vi "Main.vi"() -> ()   [LabVIEW 2017]
doc: "This Continuous Measurement sample project is based on the Queued Message Handler template.\n\nThe Event Handling Loop generates messages based on user interface actions.\n\nThe Message Handling Loop processes messages generated by the Event Handling Loop, or by other messages. There are also Acquisition and Logging message handling loop subVIs, and a chart updating loop."
uses:
  controls/UI Data.ctl
  support/libs/PMU Buffer/Buffer DATA cluster.ctl
  controls/UI State.ctl
  acquisition/Acquisition Settings.ctl
  acquisition/Acquisition State.ctl
  logging/Logging Configuration.ctl
  logging/Logging State.ctl
  support/libs/PMU Buffer/Buffer Settings.ctl
  processing/Processing Settings.ctl
  controls/Acquired Data.ctl
  <vilib>/Utility/error.llb/DialogType.ctl
  support/libs/PMU Buffer/Buffer state.ctl
  b850246f-c621-4cc8-8cdb-6c63488b8d16.vi
  d6c7b380-5ef8-42a0-a533-ce26cb609579.vi
  5953c9e4-e6ed-48ce-a3e3-f4074e595e54.vi
  308fbb3a-e3c1-4651-8528-14e79cd65b6c.vi
  e1cf4c14-b580-4597-8acf-5221adc64a8a.vi
  17f702fa-b3ef-4227-89b6-1808d4fdff79.vi
  <vilib>/S3DK/PMU Recorder Light/PRL Channel Selector.vi
  support/settings/Get Config File Path.vi
  <vilib>/Utility/xml.llb/Read From XML File.vi
  <vilib>/Utility/xml.llb/Read From XML File(string).vi
  <vilib>/Utility/xml.llb/Write to XML File.vi
  <vilib>/Utility/xml.llb/Write to XML File(string).vi
  <vilib>/Utility/error.llb/Error Cluster From Error Code.vi
  <vilib>/ErrorRing/Error Ring.xnode
  Acquisition/Acquisition.lvlib
  Logging/Logging.lvlib
  support/User Event - Stop/User Event - Stop.lvlib
  support/Message Queue/Message Queue.lvlib
  support/settings/Settings Dialog.vi
  support/settings/Settings.lvlib
  processing/Processing.lvlib
  support/libs/PMU Buffer/PMU data buffer.lvlib
  <vilib>/S3DK/PMU Recorder Light/PMU Recorder Light.lvlib
panel:
  in  "Data Selector":bool
  in  "PRL Visible":bool
  out "Processing":bool=TRUE
  out "Display":bool
  out "Acquisition":bool=TRUE
  out "Events":bool=TRUE
  out "Buffer":bool
  out "UI Control":bool
  out "Waveform Chart":dbl[](graph)
  in  "Settings":bool
  in  "Start":bool
  in  "Stop":bool
  out "Status":string
  in  "Exit":bool
  # "Continuous Measurement Data Logger"
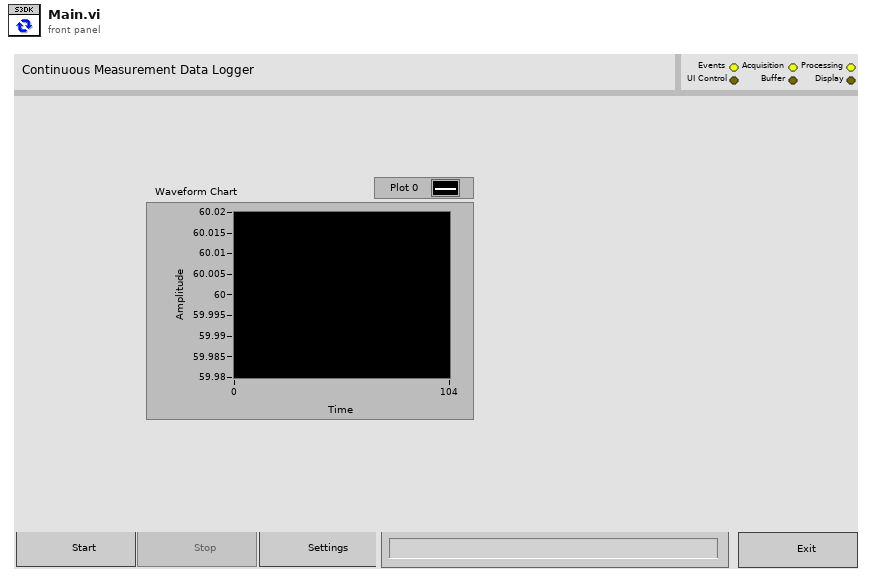
[diagram p1: front panel]
types:
  T1 = typedef "Acquired Data.ctl" = cluster{"Data":dbl[]}
  T2 = typedef "Processing.lvlib/Processing Settings.ctl" = cluster{"Settings":string, "Parameters":T3}
  T3 = typedef "PMU data buffer.lvlib/Buffer Settings.ctl" = cluster{"Index":i32, "Size":i32, "Samples":i32, "Ordered ?":bool}
  T4 = typedef "Logging.lvlib/Logging Configuration.ctl" = cluster{"Logging State":T5, "Settings":string, "Buffer":T3}
  T5 = typedef "Logging.lvlib/Logging State.ctl" = enum16{"Idle", "Logging"}
  T6 = typedef "Acquisition.lvlib/Acquisition Settings.ctl" = cluster{"Acquisition State":T7, "Settings":string, "Status":cluster{"Buffer":bool, "Config":bool, "Connect":bool}, "S3DK":cluster{"Signals":cluster{"Phasor":string[], "Analog":string[], "Digital":string[]}}}
  T7 = typedef "Acquisition.lvlib/Acquisition State.ctl" = enum16{"Idle S3DK", "Acquiring S3DK", "Idle CSV", "Acquiring CSV"}
  T8 = typedef "UI State.ctl" = enum16{"Idle", "Acquiring and Logging", "Waiting for Exit", "Waiting for Exit (Acq Stopped)", "Waiting for Exit (Log Stopped)", "Waiting for Stop", "Waiting for Stop (Acq Stopped)", "Waiting for Stop (Log Stopped)"}
  T9 = typedef "PMU data buffer.lvlib/Buffer DATA cluster.ctl" = cluster{timestamp, csg[], sgl[]}
  T10 = typedef "UI Data.ctl" = cluster{"Start Ref":refnum<vi>, "Stop Ref":refnum<vi>, "Settings Ref":refnum<vi>, "Exit Ref":refnum<vi>, "Status Ref":refnum<vi>, "Data Ref":refnum<vi>}
  T11 = cluster{"notifier out":refnum<notifier>, "notifier out":refnum<notifier>, "notifier out":refnum<notifier>}
  T12 = typedef "Message Queue.lvlib/All Message Queues.ctl" = cluster{"UI":refnum<queue>, "Acquisition":refnum<queue>, "Logging":refnum<queue>, "Processing":refnum<queue>}
  T13 = cluster{"Data Cluster":T6, "Logging Configuration":T4, "Processing Settings":T2}
  T14 = typedef "Settings.lvlib/Settings.ctl" = cluster{"Hardware Configuration":T6, "Logging Configuration":T4, "Processing Settings":T2}
  T15 = typedef "DialogType.ctl" = u16
  T16 = enum16{"Run", "Startup", "Get Status", "Pause", "Continue", "Shutdown", "Abort", "Open Panel", "Close Panel"}
  T17 = enum32{"Invalid", "Standard", "Closed", "Hidden", "Minimized", "Maximized"}
  T18 = typedef "PMU data buffer.lvlib/Buffer state.ctl" = enum16{"Init", "Change Size", "Flush", "Exit", "Add", "Get", "Hist_Toggle", "Add_Serv"}
  T19 = typedef "PMU data buffer.lvlib/Buffer DATA OUT ordered.ctl" = cluster{"Timestamp":timestamp[], "Phasor":csg[][], "Analog":sgl[][]}
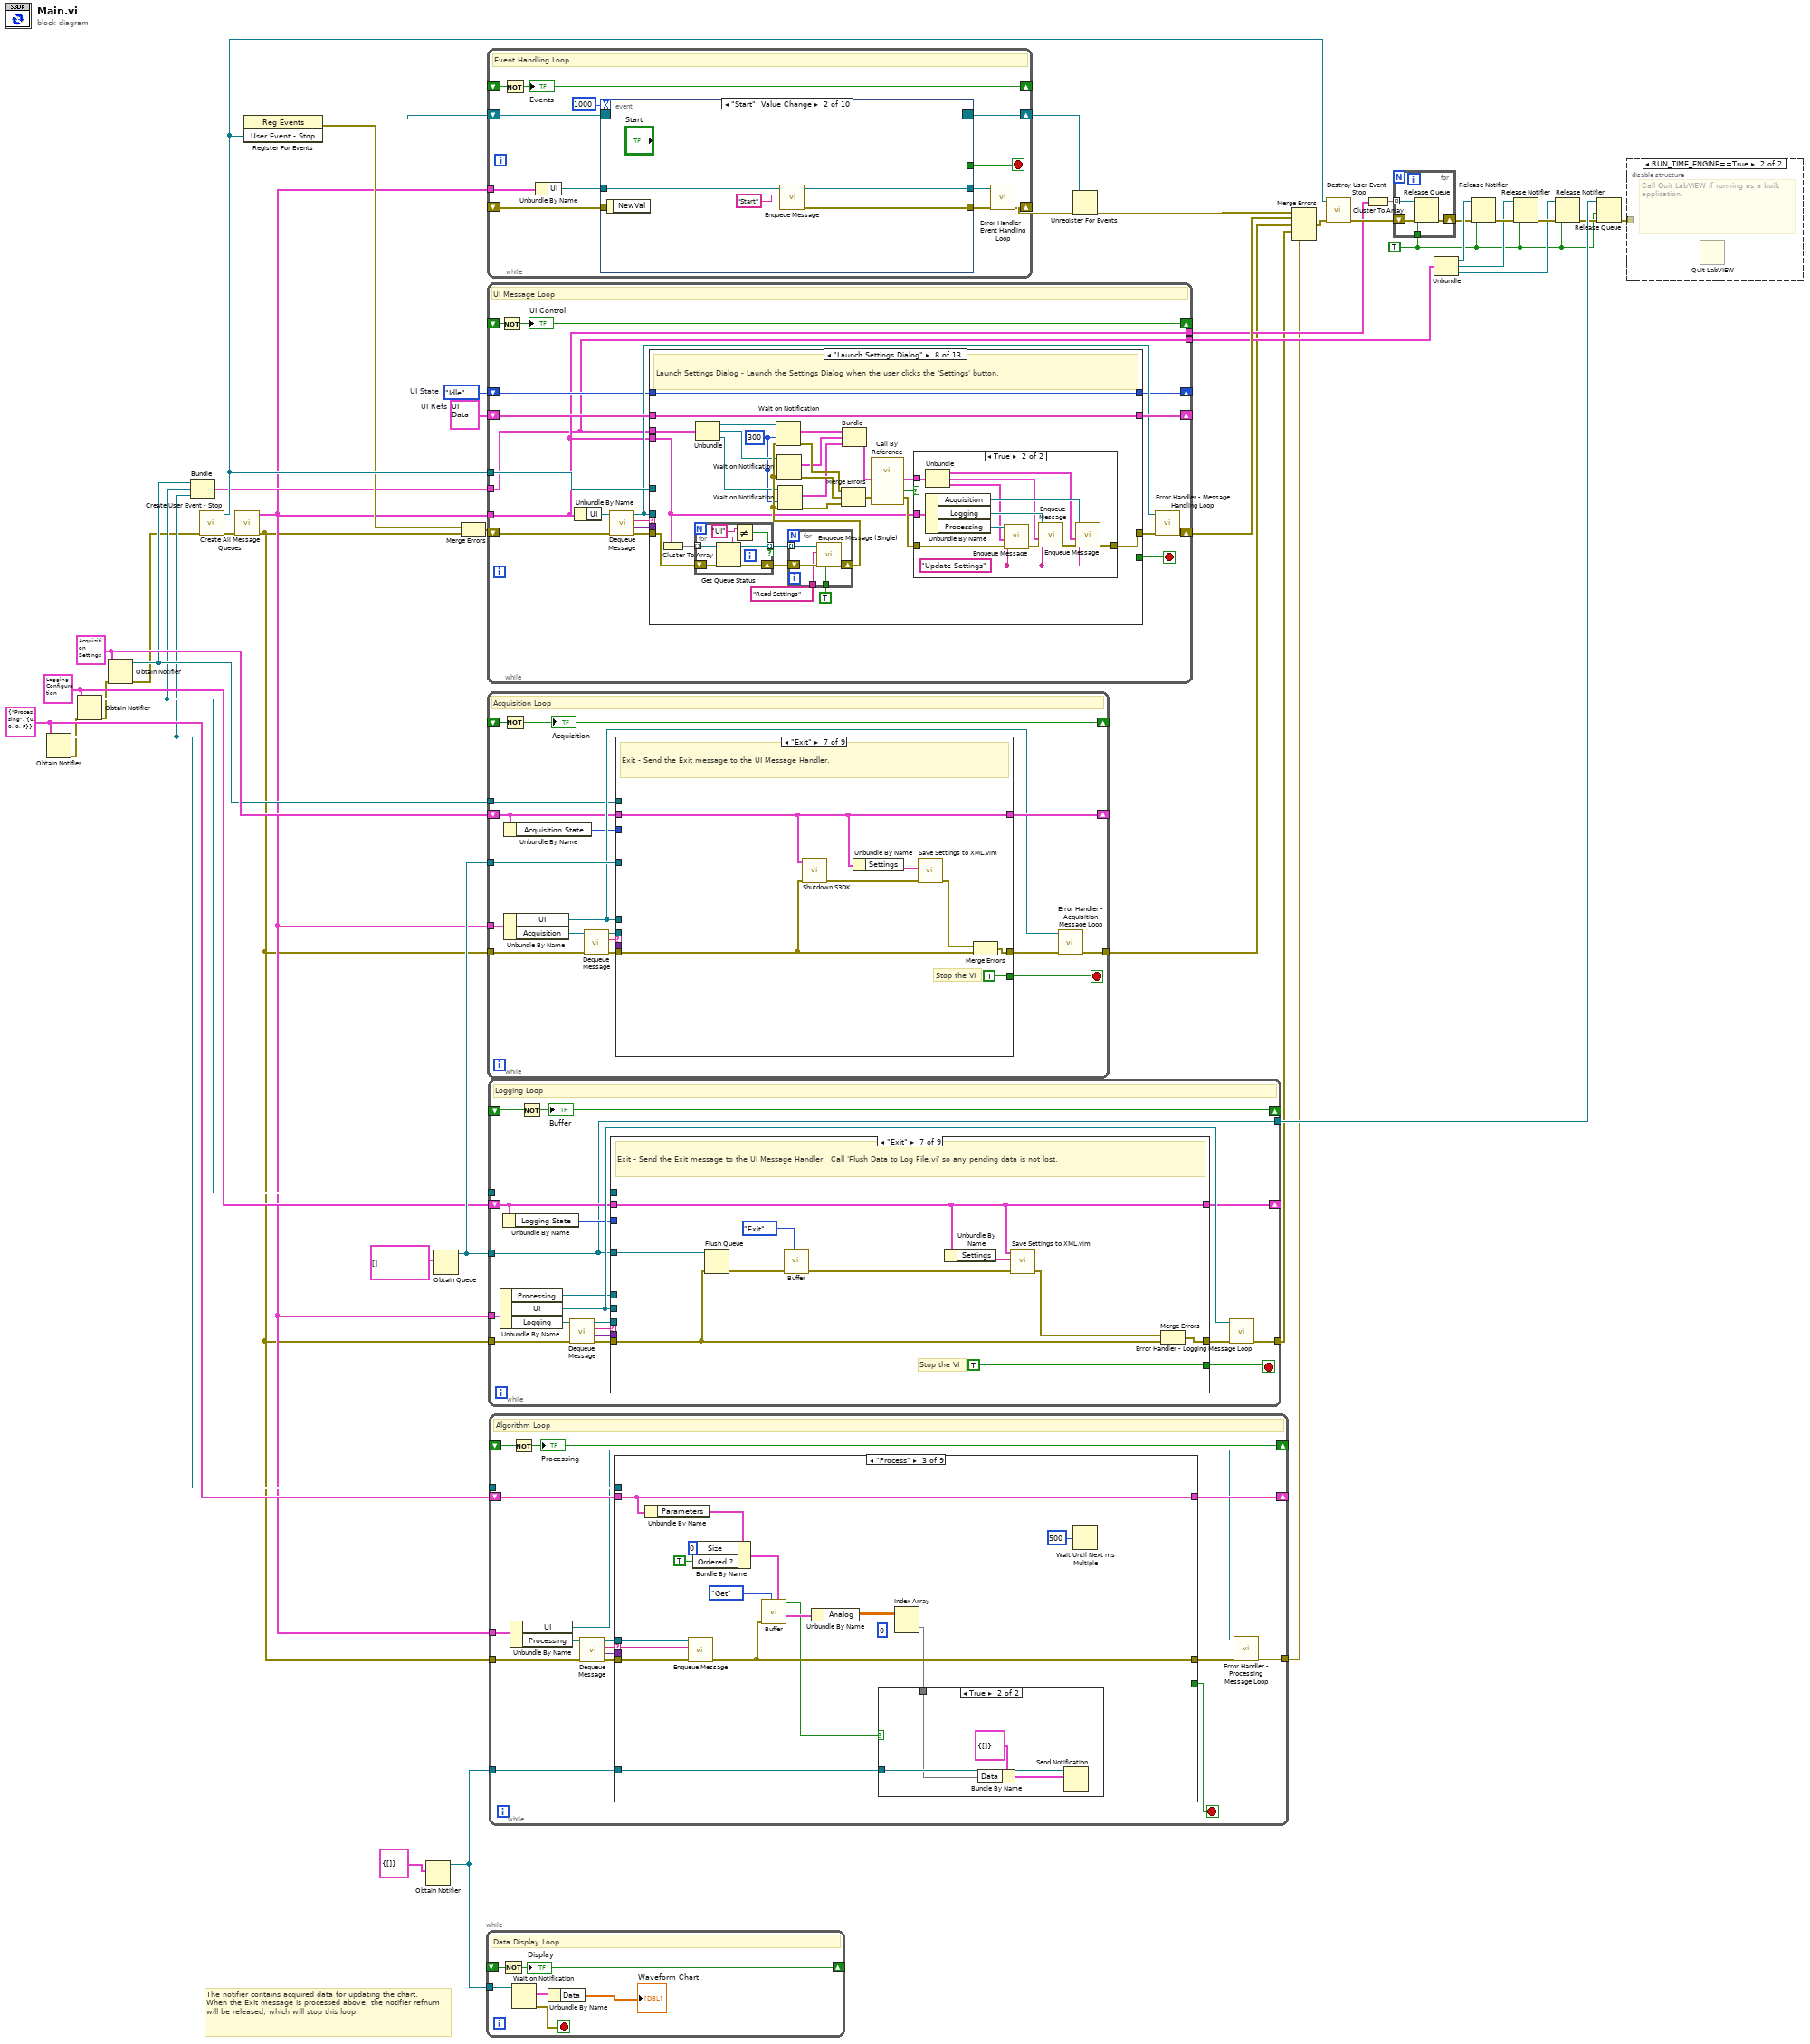
[diagram p0: block diagram]
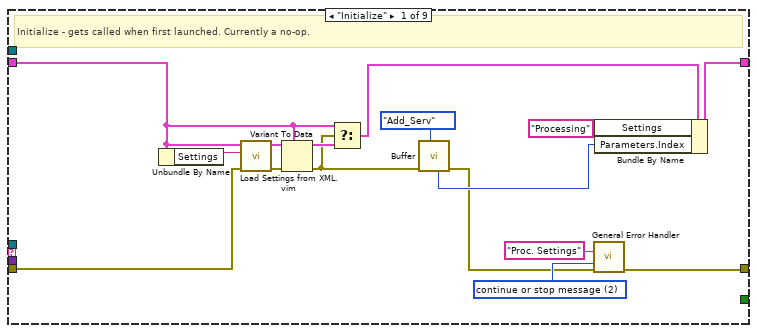
[diagram p2: hidden frame]
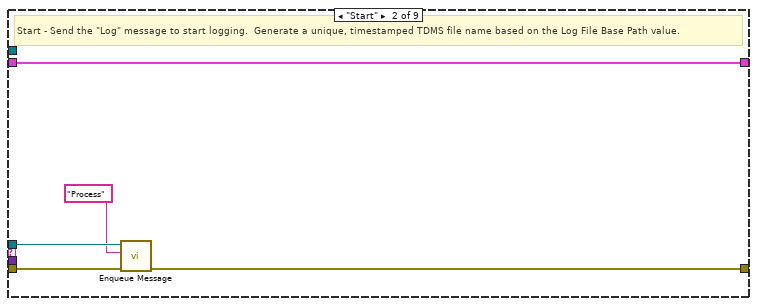
[diagram p3: hidden frame]
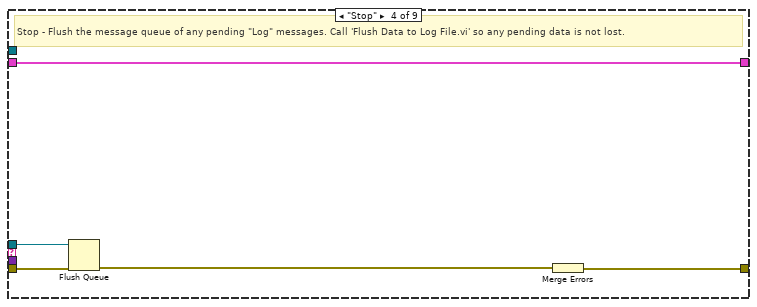
[diagram p5: hidden frame]
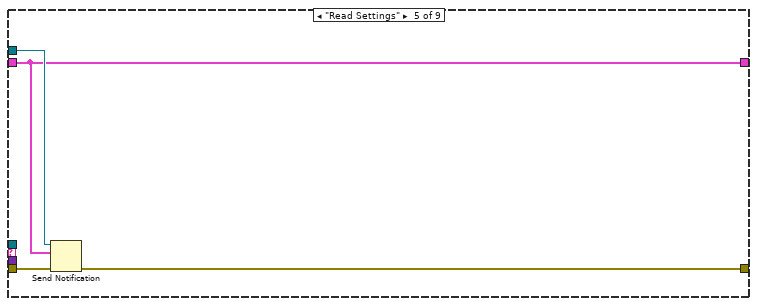
[diagram p6: hidden frame]
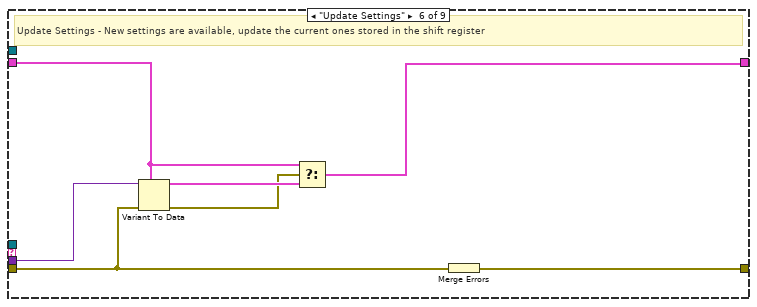
[diagram p7: hidden frame]
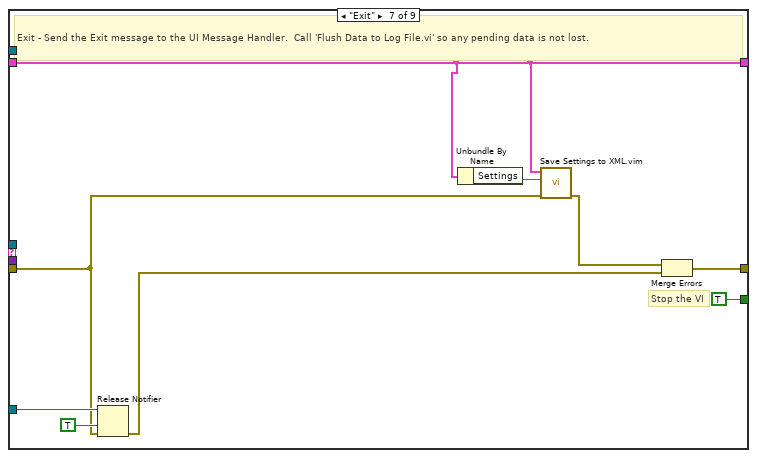
[diagram p8: hidden frame]
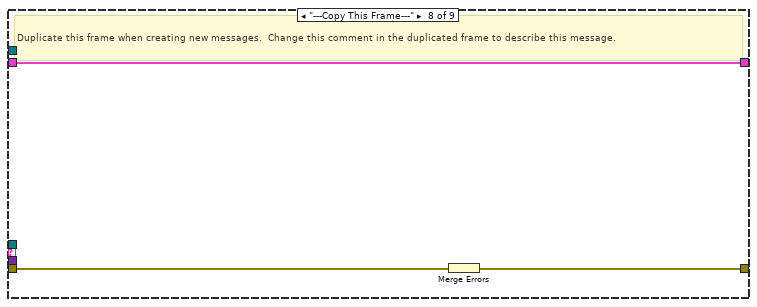
[diagram p9: hidden frame]
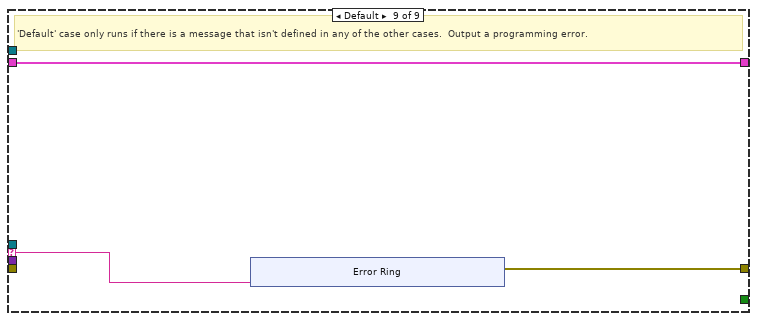
[diagram p10: hidden frame]
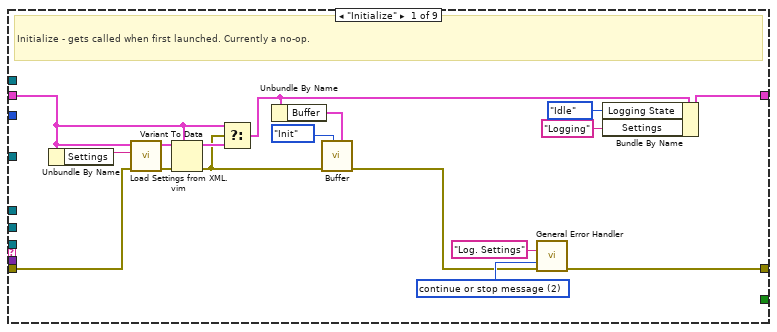
[diagram p11: hidden frame]
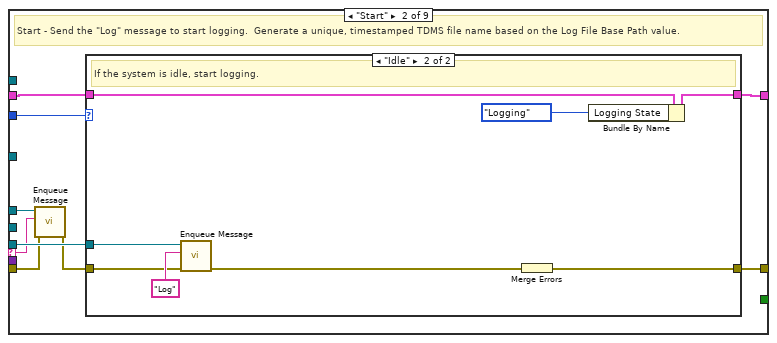
[diagram p12: hidden frame]
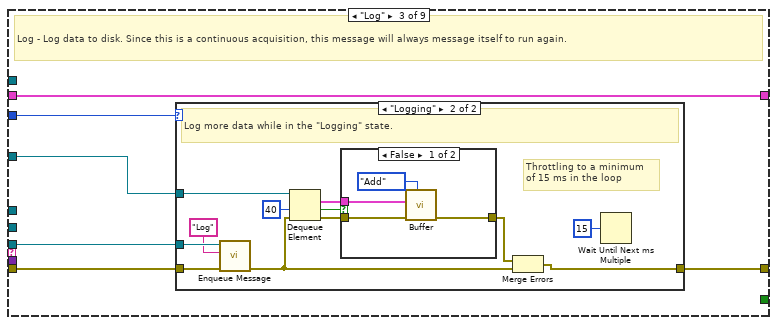
[diagram p14: hidden frame]
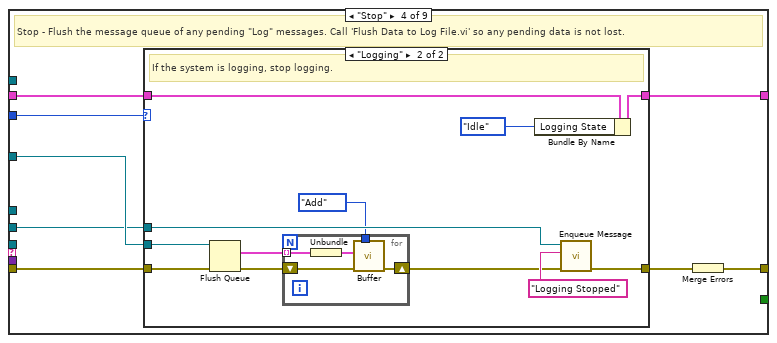
[diagram p17: hidden frame]
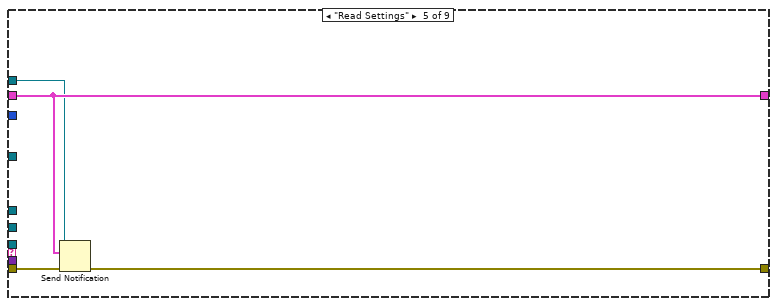
[diagram p19: hidden frame]
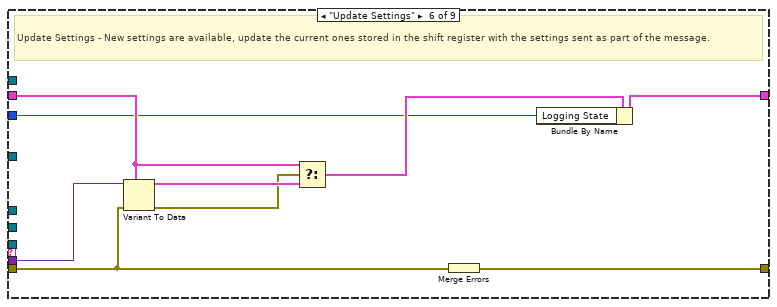
[diagram p20: hidden frame]
diagram:
  w26 = T2 {"Settings"="Processing", "Parameters"={"Index"=0, "Size"=0, "Samples"=0, "Ordered ?"=FALSE}} ("Processing Settings")
  w6 = TRUE ("force destroy? (F)")
  w27 = T4 {"Logging State"=enum."Idle", "Settings"="Logging", "Buffer"={"Index"=0, "Size"=15000, "Samples"=0, "Ordered ?"=FALSE}} ("Logging Configuration")
  w28 = T6 {"Acquisition State"=enum."Idle S3DK", "Settings"="Acquisition", "Status"={"Buffer"=FALSE, "Config"=FALSE, "Connect"=FALSE}, "S3DK"={"Signals"={"Phasor"=[], "Analog"=[], "Digital"=[]}}} ("Data Cluster")
  w41 = UI_State."Idle"  # UI State
  w42 = T10 {"Start Ref"=refnum, "Stop Ref"=refnum, "Settings Ref"=refnum, "Exit Ref"=refnum, "Status Ref"=refnum, "Data Ref"=refnum}  # UI Refs
  # "The notifier contains acquired data for updating the chart. When the Exit message is processed above, the notifier refnum will be released, which will stop this loop."
  n1 = Obtain Notifier(notification data type=w26) -> (notifier out=w23:refnum<notifier>, error out=w20:errorcluster)  [unwired: 3 in, 1 out]
  n2 = Obtain Notifier(notification data type=w27, error in (no error)=w20) -> (notifier out=w24:refnum<notifier>, error out=w21:errorcluster)  [unwired: 2 in, 1 out]
  n3 = Obtain Notifier(notification data type=w28, error in (no error)=w21) -> (notifier out=w25:refnum<notifier>, error out=w22:errorcluster)  [unwired: 2 in, 1 out]
  n4 = Bundle("notifier out"=w25, "notifier out"=w24, "notifier out"=w23) -> (w19:T11)  [unwired: 1 in]
  n5 = call "Create User Event - Stop.vi"("error in (no error)"=w22) -> ("error out"=w44:errorcluster, "User Event - Stop"=w38:refnum<user-event>)  [unwired: 9 in]
  n6 = call "Create All Message Queues.vi"("error in (no error)"=w44) -> ("error out"=w4:errorcluster, "Message Queues out"=w17:T12)  [unwired: 9 in]
  n7 = register-events(w38) -> (reference out=w39:refnum<event-registration>, error out=w36:errorcluster)  [unwired: 2 in]
  n8 = Obtain Notifier(notification data type=T1 {"Data"=[]} ("Display Data")) -> (notifier out=w29:refnum<notifier>)  [unwired: 3 in, 2 out]
  n9 = Obtain Queue(element data type=T9[] []) -> (queue out=w35:refnum<queue>)  [unwired: 4 in, 2 out]
  n10 = Merge Errors(w36, w4) -> (w37:errorcluster)
  n11 = while "Data Display Loop" {
    tunnel: w29 -> [w51]
    shift-right: [w49] -> _
    shift-left: _ -> [w48]
    stop <- w50 stop-if-true
    # "Data Display Loop"
    n12 = Not(x=w48) -> (.not. x?=w49:bool)
    "Display" <- w49
    n13 = Wait on Notification(notifier=w51) -> (notification=w47:T1, error out=w50:errorcluster)  [unwired: 3 in, 2 out]
    n14 = Unbundle By Name(w47) -> ("Data"=→"Waveform Chart":dbl[])
  }
  n15 = while {
    tunnel: w38 -> [w68]
    shift-right: [w63] -> _
    shift-left: w42 -> [w64]
    shift-right: [w58] -> _
    shift-left: w41 -> [w59]
    tunnel: w17 -> [w53]
    tunnel: w19 -> [w52]
    shift-right: [w54] -> _
    shift-left: _ -> [w55]
    tunnel: [w53] -> w16
    tunnel: [w52] -> w12
    shift-right: [w62] -> w33
    shift-left: w37 -> [w67]
    stop <- w69 stop-if-true
    # "UI Message Loop"
    n16 = Not(x=w55) -> (.not. x?=w54:bool)
    "UI Control" <- w54
    n17 = Unbundle By Name(w53) -> ("UI"=w57:refnum<queue>)
    n18 = call "Dequeue Message.vi"("error in (no error)"=w67, "Message Queue"=w57) -> ("error out"=w56:errorcluster, "Message Data"=w65:variant, "Message"=w66:string, "dup Message Queue"=w60:refnum<queue>)  [unwired: 6 in]
    n19 = case "Message Cases" shown="\"Launch Settings Dialog\"" w66 {
      selector: w66 -> [_ _ _ _ _ _ _ _ _ _ _ _ w313]
      tunnel: w60 -> [w71 _ _ w122 _ w146 w170 _ _ w256 _ _ _]
      tunnel: w56 -> [w72 w92 w99 w121 w140 w147 w171 w192 w245 w255 w280 w311 _]
      tunnel: [w79 w92 w100 w106 w141 w144 w168 w214 w248 w254 w293 w310 w312] -> w61
      tunnel: [_ _ _ _ _ _ _ _ _ _ TRUE _ _] -> w69
      tunnel: w65 -> [_ _ w98 _ _ _ _ _ w249 _ w289 _ _]
      tunnel: w68 -> [_ _ _ _ _ _ _ _ _ _ w294 _ _]
      tunnel: w64 -> [w76 w91 w94 w118 w139 w149 w173 w216 w252 w258 w292 w309 w315]
      tunnel: [w76 w89 w94 w118 w139 w149 w173 w216 w252 w258 w292 w309 w315] -> w63
      tunnel: w59 -> [_ _ w93 _ w127 w148 w172 w215 w247 w257 _ w308 w314]
      tunnel: [UI_State."Idle" ("UI State") UI_State."Idle" ("UI State") w93 UI_State."Acquiring and Logging" ("UI State") w128 w145 w169 w215 w247 w253 UI_State."Idle" ("UI State") w308 w314] -> w58
      tunnel: w53 -> [_ _ _ w101 w126 _ _ w196 _ _ w284 _ _]
      tunnel: w52 -> [_ _ _ _ _ _ _ w210 _ _ _ _ _]
      frame "Initialize" {
        # "Initialize - Get configuration settings, then message the UI to initialize, and broadcast the settings to the other message loops."
        n20 = call-poly "Enqueue Message.vi"("error in (no error)"=w72, "Message"="Init UI Refs", "Message Queue"=w71) -> ("error out"=w73:errorcluster, "dup Message Queue"=w74:refnum<queue>)  [unwired: 7 in]
        n21 = call-poly "Enqueue Message.vi"("error in (no error)"=w73, "Message Data"="Ready..." ("Ready..."), "Message"="Update Status", "Message Queue"=w74) -> ("error out"=w79:errorcluster)  [unwired: 6 in, 1 out]
      }
      frame "Init UI Refs" {
        # "Enable: Start, Exit, Settings\nDisable: Stop"
        # "Init UI Refs - Store control references for UI controls.  Also enable/disable controls appropriately."
        n22 = control-ref of="Start"() -> (w83:refnum<vi>)
        n23 = control-ref of="Stop"() -> (w84:refnum<vi>)
        n24 = control-ref of="Settings"() -> (w82:refnum<vi>)
        n25 = control-ref of="Exit"() -> (w81:refnum<vi>)
        n26 = control-ref of="Status"() -> (w90:refnum<vi>)
        n27 = Bundle By Name(cluster=w91, "Start Ref"=w83, "Stop Ref"=w84, "Settings Ref"=w82, "Exit Ref"=w81, "Status Ref"=w90) -> (w89:T10)
        n28 = Build Array(w83, w82, w81) -> (w87:refnum<vi>[])
        n29 = Build Array(w84) -> (w86:refnum<vi>[])
        n30 = call "Set Enable State on Multiple Controls.vi"("Enable?"=TRUE, "Controls"=w87) -> ()  [unwired: 10 in]
        n31 = call "Set Enable State on Multiple Controls.vi"("Enable?"=FALSE, "Controls"=w86) -> ()  [unwired: 10 in]
      }
      frame "Update Status" {
        # "Update Status - Convert the message data to a string to display in the Status indicator."
        n32 = Variant To Data(error in=w99, type="", Variant=w98) -> (data=→"Status":string, error out=w96:errorcluster)
        n33 = Merge Errors(w96) -> (w100:errorcluster)
      }
      frame "Start" {
        # "Message Acquisition and Logging loops to start."
        # "Enable: Stop\nDisable: Start, Exit, Settings"
        # "Start - Enable/Disable buttons appropriately for an acquisition that has started, and update status display."
        n34 = Unbundle By Name(w118) -> ("Stop Ref"=w113:refnum<vi>, "Start Ref"=w112:refnum<vi>, "Exit Ref"=w111:refnum<vi>, "Settings Ref"=w110:refnum<vi>)
        n35 = call-poly "Enqueue Message.vi"("error in (no error)"=w121, "Message Data"="Acquiring and Logging..." ("Acquiring and Logging..."), "Message"="Update Status", "Message Queue"=w122) -> ("error out"=w109:errorcluster)  [unwired: 6 in, 1 out]
        n36 = Build Array(w112, w111, w110) -> (w116:refnum<vi>[])
        n37 = Build Array(w113) -> (w115:refnum<vi>[])
        n38 = Unbundle By Name(w101) -> ("Acquisition"=w102:refnum<queue>)
        n39 = call "Set Enable State on Multiple Controls.vi"("Enable?"=TRUE, "Controls"=w115) -> ()  [unwired: 10 in]
        n40 = call "Set Enable State on Multiple Controls.vi"("Enable?"=FALSE, "Controls"=w116) -> ()  [unwired: 10 in]
        n41 = call-poly "Enqueue Message.vi"("error in (no error)"=w109, "Message"="Start", "Message Queue"=w102) -> ("error out"=w107:errorcluster)  [unwired: 7 in, 1 out]
        n42 = Unbundle By Name(w101) -> ("Logging"=w103:refnum<queue>)
        n43 = call-poly "Enqueue Message.vi"("error in (no error)"=w107, "Message"="Start", "Message Queue"=w103) -> ("error out"=w106:errorcluster)  [unwired: 7 in, 1 out]
      }
      frame "Stop" {
        w123 = "Stop" ("Message")
        # "Message Acquisition and Logging loops to stop"
        # "Enable: Start, Exit, Settings\nDisable: Stop"
        # "Stop - Enable/Disable buttons appropriately for an acquisition that has stopped, and update status display."
        n44 = Unbundle By Name(w126) -> ("Acquisition"=w124:refnum<queue>)
        n45 = Unbundle By Name(w139) -> ("Stop Ref"=w134:refnum<vi>, "Start Ref"=w133:refnum<vi>, "Exit Ref"=w132:refnum<vi>, "Settings Ref"=w131:refnum<vi>)
        n46 = call-poly "Enqueue Message.vi"("error in (no error)"=w140, "Message"=w123, "Message Queue"=w124) -> ("error out"=w130:errorcluster)  [unwired: 7 in, 1 out]
        n47 = Unbundle By Name(w126) -> ("Logging"=w125:refnum<queue>)
        n48 = Build Array(w133, w132, w131) -> (w137:refnum<vi>[])
        n49 = Build Array(w134) -> (w136:refnum<vi>[])
        n50 = call-poly "Enqueue Message.vi"("error in (no error)"=w130, "Message"=w123, "Message Queue"=w125) -> ("error out"=w129:errorcluster)  [unwired: 7 in, 1 out]
        n51 = call "Set Enable State on Multiple Controls.vi"("Enable?"=FALSE, "Controls"=w136) -> ()  [unwired: 10 in]
        n52 = call "Set Enable State on Multiple Controls.vi"("Enable?"=TRUE, "Controls"=w137) -> ()  [unwired: 10 in]
        n53 = Merge Errors(w129) -> (w141:errorcluster)
        n54 = case shown="Default" w127 {
          selector: w127 -> [w142 _]
          tunnel: [w142 UI_State."Waiting for Stop" ("UI State")] -> w128
          frame "Waiting for Exit" {
          }
          frame Default {
          }
        }
      }
      frame "Acquisition Stopped" {
        # "Logic for determining what action to take when the acquisition has stopped."
        n55 = case shown="\"Waiting for Stop (Log Stopped)\"" w148 {
          selector: w148 -> [w151 _ _ _ _]
          tunnel: w147 -> [w150 w153 w155 w161 w167]
          tunnel: w146 -> [_ _ _ w159 w164]
          tunnel: [w151 UI_State."Waiting for Exit (Acq Stopped)" ("UI State") UI_State."Waiting for Stop (Acq Stopped)" ("UI State") UI_State."Idle" ("UI State") UI_State."Idle" ("UI State")] -> w145
          tunnel: [w150 w153 w155 w160 w165] -> w144
          frame Default {
          }
          frame "Waiting for Exit", "Waiting for Exit (Acq Stopped)" {
          }
          frame "Waiting for Stop", "Waiting for Stop (Acq Stopped)" {
          }
          frame "Waiting for Exit (Log Stopped)" {
            # "If we are waiting to exit, and the logging has already stopped, then the \"Acquisition Stopped\" message indicates that it is time to exit."
            n56 = call-poly "Enqueue Message.vi"("Priority Message? (F)"=TRUE, "error in (no error)"=w161, "Message"="Exit", "Message Queue"=w159) -> ("error out"=w160:errorcluster)  [unwired: 6 in, 1 out]
          }
          frame "Waiting for Stop (Log Stopped)" {
            # "If we are waiting to stop, and the logging has already stopped, then the \"Acquisition Stopped\" message indicates that it is time to stop."
            n57 = call-poly "Enqueue Message.vi"("error in (no error)"=w167, "Message Data"="Ready..." ("Ready..."), "Message"="Update Status", "Message Queue"=w164) -> ("error out"=w165:errorcluster)  [unwired: 6 in, 1 out]
          }
        }
      }
      frame "Logging Stopped" {
        # "Logic for determining what action to take when the logging has stopped."
        n58 = case shown="\"Waiting for Stop (Acq Stopped)\"" w172 {
          selector: w172 -> [w175 _ _ _ _]
          tunnel: w171 -> [w174 w177 w179 w185 w188]
          tunnel: w170 -> [_ _ _ w183 w187]
          tunnel: [w175 UI_State."Waiting for Exit (Log Stopped)" ("UI State") UI_State."Waiting for Stop (Log Stopped)" ("UI State") UI_State."Idle" ("UI State") UI_State."Idle" ("UI State")] -> w169
          tunnel: [w174 w177 w179 w184 w186] -> w168
          frame Default {
          }
          frame "Waiting for Exit", "Waiting for Exit (Log Stopped)" {
          }
          frame "Waiting for Stop", "Waiting for Stop (Log Stopped)" {
          }
          frame "Waiting for Exit (Acq Stopped)" {
            # "If we are waiting to exit, and the acquisition has already stopped, then the \"Logging Stopped\" message indicates that it is time to exit."
            n59 = call-poly "Enqueue Message.vi"("Priority Message? (F)"=TRUE, "error in (no error)"=w185, "Message"="Exit", "Message Queue"=w183) -> ("error out"=w184:errorcluster)  [unwired: 6 in, 1 out]
          }
          frame "Waiting for Stop (Acq Stopped)" {
            # "If we are waiting to stop, and the acquisition has already stopped, then the \"Logging Stopped\" message indicates that it is time to stop."
            n60 = call-poly "Enqueue Message.vi"("error in (no error)"=w188, "Message Data"="Ready..." ("Ready..."), "Message"="Update Status", "Message Queue"=w187) -> ("error out"=w186:errorcluster)  [unwired: 6 in, 1 out]
          }
        }
      }
      frame "Launch Settings Dialog" {
        w198 = 300 ("timeout in ms (-1)")
        # "Launch Settings Dialog - Launch the Settings Dialog when the user clicks the 'Settings' button."
        n61 = Cluster To Array(cluster=w196) -> (array=w195:refnum<queue>[])
        n62 = for {
          tunnel: w195 -> [w225] mode=indexing
          tunnel: [w224] -> w194 mode=indexing if=w221
          shift-right: [w220] -> w193
          shift-left: w192 -> [w219]
          n63 = Get Queue Status(queue=w225, error in (no error)=w219) -> (queue out=w224:refnum<queue>, queue name=w223:string, error out=w220:errorcluster)  [unwired: 1 in, 5 out]
          n64 = Not Equal?(x="UI" ("y"), y=w223) -> (x != y?=w221:bool)
        }
        n65 = Unbundle(w210) -> ("notifier out"=w209:refnum<notifier>, "notifier out"=w200:refnum<notifier>, "notifier out"=w199:refnum<notifier>)
        n66 = for {
          tunnel: TRUE -> [w230]
          shift-right: [w228] -> w208
          shift-left: w193 -> [w229]
          tunnel: w194 -> [w227] mode=indexing
          tunnel: "Read Settings" ("Message") -> [w226]
          n67 = call "Enqueue Message (Single).vi"("Priority Message? (F)"=w230, "error in (no error)"=w229, "Message"=w226, "Message Queue"=w227) -> ("error out"=w228:errorcluster)  [unwired: 6 in, 1 out]
        }
        n68 = Wait on Notification(notifier=w209, timeout in ms (-1)=w198, error in (no error)=w208) -> (notification=w204:T6, error out=w205:errorcluster)  [unwired: 1 in, 2 out]
        n69 = Wait on Notification(notifier=w200, timeout in ms (-1)=w198, error in (no error)=w208) -> (notification=w203:T4, error out=w206:errorcluster)  [unwired: 1 in, 2 out]
        n70 = Wait on Notification(notifier=w199, timeout in ms (-1)=w198, error in (no error)=w208) -> (notification=w202:T2, error out=w207:errorcluster)  [unwired: 1 in, 2 out]
        n71 = Merge Errors(w205, w206, w207) -> (w211:errorcluster)
        n72 = Bundle("Data Cluster"=w204, "Logging Configuration"=w203, "Processing Settings"=w202) -> (w201:T13)  [unwired: 1 in]
        n73 = call-by-ref "?"("error in (no error)"=w211, "Settings in"=w201) -> ("error out"=w217:errorcluster, "Changed?"=w218:bool, "Settings out"=w197:T14)  [unwired: 8 in, 3 out]
        n74 = case shown="True" w218 {
          tunnel: w217 -> [w231 w244]
          tunnel: [w231 w239] -> w214
          tunnel: w197 -> [_ w243]
          tunnel: w196 -> [_ w242]
          frame False {
          }
          frame True {
            w232 = "Update Settings" ("Message")
            n75 = Unbundle(w243) -> ("Hardware Configuration"=w233:T6, "Logging Configuration"=w234:T4, "Processing Settings"=w235:T2)
            n76 = Unbundle By Name(w242) -> ("Acquisition"=w236:refnum<queue>, "Logging"=w237:refnum<queue>, "Processing"=w238:refnum<queue>)
            n77 = call-poly "Enqueue Message.vi"("error in (no error)"=w244, "Message Data"=w235, "Message"=w232, "Message Queue"=w238) -> ("error out"=w241:errorcluster)  [unwired: 6 in, 1 out]
            n78 = call-poly "Enqueue Message.vi"("error in (no error)"=w241, "Message Data"=w234, "Message"=w232, "Message Queue"=w237) -> ("error out"=w240:errorcluster)  [unwired: 6 in, 1 out]
            n79 = call-poly "Enqueue Message.vi"("error in (no error)"=w240, "Message Data"=w233, "Message"=w232, "Message Queue"=w236) -> ("error out"=w239:errorcluster)  [unwired: 6 in, 1 out]
          }
        }
      }
      frame "Error" {
        # "Error - Display an error dialog. This message is sent by the \"Error Handler\" VIs at the end of other loops in this application."
        n80 = Variant To Data(error in=w245, type=errorcluster {"status"=FALSE, "code"=0, "source"=""} ("error constant"), Variant=w249) -> (data=w246:errorcluster, error out=w250:errorcluster)
        n81 = call <vilib>:"Simple Error Handler.vi"("error in (no error)"=w246) -> ()  [unwired: 4 in, 5 out]
        n82 = Merge Errors(w250) -> (w248:errorcluster)
      }
      frame "Confirm Quit" {
        # "Confirm Quit - Message that can confirm whether or not the user wants to exit the application."
        n83 = case shown="\"Acquiring and Logging\"" w257 {
          tunnel: w256 -> [w264 w268]
          tunnel: w255 -> [w263 w267]
          tunnel: [w262 w266] -> w254
          tunnel: [UI_State."Idle" ("UI State") w265] -> w253
          frame Default {
            # "If 'Confirm Quit' comes in while the system is idle, there is no need for a confirmation message."
            n84 = call-poly "Enqueue Message.vi"("Priority Message? (F)"=TRUE, "error in (no error)"=w263, "Message"="Exit", "Message Queue"=w264) -> ("error out"=w262:errorcluster)  [unwired: 6 in, 1 out]
          }
          frame "Acquiring and Logging" {
            n85 = Two Button Dialog(message="Are you sure you want to quit while the acquisition is running?" ("Confirm Quit Message"), 1:"No" ("No"), 2:"Yes" ("Yes")) -> (T button?=w269:bool)
            n86 = case shown="True" w269 {
              tunnel: w268 -> [_ w278]
              tunnel: w267 -> [w274 w279]
              tunnel: [w274 w277] -> w266
              tunnel: [UI_State."Acquiring and Logging" ("UI State") UI_State."Waiting for Exit" ("UI State")] -> w265
              frame False {
                # "User did not want to quit."
              }
              frame True {
                n87 = call-poly "Enqueue Message.vi"("error in (no error)"=w279, "Message"="Stop", "Message Queue"=w278) -> ("error out"=w277:errorcluster)  [unwired: 7 in, 1 out]
              }
            }
          }
        }
      }
      frame "Exit" {
        # "Popup an error dialog if 'Exit' was called as a result of an error."
        # "Stop the VI"
        # "Exit - Send Exit messages to the Acquisition and Logging loops, and fire the user event to stop the Event Handling Loop."
        n88 = Cluster To Array(cluster=w284) -> (array=w283:refnum<queue>[])
        n89 = for {
          tunnel: w283 -> [w302] mode=indexing
          tunnel: [w301] -> w282 mode=indexing if=w298
          shift-right: [w297] -> w281
          shift-left: w280 -> [w296]
          n90 = Get Queue Status(queue=w302, error in (no error)=w296) -> (queue out=w301:refnum<queue>, queue name=w300:string, error out=w297:errorcluster)  [unwired: 1 in, 5 out]
          n91 = Not Equal?(x="UI" ("y"), y=w300) -> (x != y?=w298:bool)
        }
        n92 = Variant To Data(type=errorcluster {"status"=FALSE, "code"=0, "source"=""} ("error constant"), Variant=w289) -> (data=w288:errorcluster)  [unwired: 1 in, 1 out]
        n93 = call <vilib>:"Simple Error Handler.vi"("error in (no error)"=w288) -> ()  [unwired: 4 in, 5 out]
        n94 = for {
          tunnel: TRUE ("Priority Message? (F)") -> [w307]
          tunnel: "Exit" ("Message") -> [w305]
          tunnel: w282 -> [w304] mode=indexing
          shift-right: [w303] -> w285
          shift-left: w281 -> [w306]
          n95 = call-poly "Enqueue Message.vi"("Priority Message? (F)"=w307, "error in (no error)"=w306, "Message"=w305, "Message Queue"=w304) -> ("error out"=w303:errorcluster)  [unwired: 6 in, 1 out]
        }
        n96 = call "Fire User Event - Stop.vi"("error in (no error)"=w285, "User Event - Stop"=w294) -> ("error out"=w293:errorcluster)  [unwired: 9 in]
      }
      frame "---Copy This Frame---" {
        # "Duplicate this frame when creating new messages.  Change this comment in the duplicated frame to describe this message."
        n97 = Merge Errors(w311) -> (w310:errorcluster)
      }
      frame Default {
        # "'Default' case only runs if there is a message that isn't defined in any of the other cases.  Output a programming error."
        n98 = xnode "Error Ring"("parameter 0"=w313) -> ("error out"=w312:errorcluster)
      }
    }
    n99 = call "Error Handler - Message Handling Loop.vi"("error in (no error)"=w61, "Message Queue"=w60) -> ("dup error in"=w62:errorcluster)  [unwired: 8 in, 1 out]
  }
  n100 = while {
    shift-right: [w340] -> _
    shift-left: w28 -> [w326]
    tunnel: w35 -> [w334]
    tunnel: w17 -> [w331]
    shift-right: [w327] -> _
    shift-left: _ -> [w328]
    tunnel: w25 -> [w324]
    tunnel: w4 -> [w338]
    tunnel: [w323] -> w5
    stop <- w339 stop-if-true
    # "Acquisition Loop"
    n101 = Not(x=w328) -> (.not. x?=w327:bool)
    "Acquisition" <- w327
    n102 = Unbundle By Name(w326) -> ("Acquisition State"=w325:T7)
    n103 = Unbundle By Name(w331) -> ("UI"=w330:refnum<queue>, "Acquisition"=w329:refnum<queue>)
    n104 = call "Dequeue Message.vi"("error in (no error)"=w338, "Message Queue"=w329) -> ("error out"=w337:errorcluster, "Message Data"=w335:variant, "Message"=w336:string, "dup Message Queue"=w332:refnum<queue>)  [unwired: 6 in]
    n105 = case "Message Cases" shown="\"Exit\"" w336 {
      selector: w336 -> [_ _ w379 _ _ _ _ _ w445]
      tunnel: w332 -> [_ w357 w385 _ _ _ _ _ _]
      tunnel: w337 -> [w345 w358 w384 w407 w425 w428 w436 w444 _]
      tunnel: [w349 w360 w386 w408 w424 w434 w440 w442 w446] -> w333
      tunnel: w326 -> [w343 w359 w382 w405 w423 w430 w438 w443 w447]
      tunnel: [w354 w356 w383 w402 w423 w427 w438 w443 w447] -> w340
      tunnel: [_ _ _ _ _ _ TRUE _ _] -> w339
      tunnel: w335 -> [_ _ _ _ _ w433 _ _ _]
      tunnel: w330 -> [_ _ _ w403 _ _ _ _ _]
      tunnel: w334 -> [_ _ w381 _ _ _ _ _ _]
      tunnel: w325 -> [_ w355 w380 w404 _ w426 _ _ _]
      tunnel: w324 -> [_ _ _ _ w422 _ _ _ _]
      frame "Initialize" {
        w347 = T15 2 items=["no dialog", "OK message", "continue or stop message", "OK message + warnings", "continue/stop + warnings"] ("type of dialog (OK msg:1)")
        # "Initialize  - Initialize is currently a no-op.  The hardware initialization takes place in the 'Start' message."
        n106 = Unbundle By Name(w343) -> ("Settings"=w342:string)
        n107 = call "Load Settings from XML.vim"("error in (no error)"=w345, "Settings File Name"=w342, "Settings In"=w343) -> ("error out"=w346:errorcluster, "Settings Out"=w344:T6)  [unwired: 7 in]
        n108 = Variant To Data(error in=w346, type=w343, Variant=w344) -> (data=w352:T6, error out=w350:errorcluster)
        n109 = Select(t=w343, s=w350, f=w352) -> (s? t:f=w351:T6)
        n110 = call <vilib>:"General Error Handler.vi"("[error source] (\" \")"="Acq. Settings" ("[error source] (\" \")"), "type of dialog (OK msg:1)"=w347, "error in (no error)"=w350) -> ("error out"=w349:errorcluster)  [unwired: 8 in, 4 out]
        n111 = Bundle By Name(cluster=w351, "Acquisition State"=Acquisition_State."Idle S3DK", "Settings"="Acquisition") -> (w354:T6)
      }
      frame "Start" {
        # "Start - Configure and start the acquisition."
        n112 = case shown="\"Idle S3DK\"" w355 {
          tunnel: [w361 w374 w376 w378] -> w360
          tunnel: w359 -> [w362 w373 w375 w377]
          tunnel: w358 -> [w361 w372 w376 w378]
          tunnel: w357 -> [_ w370 _ _]
          tunnel: [w362 w364 w375 w377] -> w356
          frame "Acquiring S3DK" {
            # "The system is already acquiring. Ignore the \"Start\" message."
          }
          frame "Idle S3DK" {
            # "If the system is idle, start the acquisition."
            n113 = call "Initialize Data Acquisition.vi"("error in (no error)"=w372, "Hardware Resources in"=w373) -> ("error out"=w369:errorcluster, "Hardware Resources out"=w367:T6)  [unwired: 8 in]
            n114 = call-poly "Enqueue Message.vi"("error in (no error)"=w372, "Message"="Acquire", "Message Queue"=w370) -> ("error out"=w371:errorcluster)  [unwired: 7 in, 1 out]
            n115 = call "Configure Hardware.vi"("error in (no error)"=w369, "Hardware Resources in"=w367) -> ("error out"=w368:errorcluster, "Hardware Resources out"=w366:T6)  [unwired: 8 in]
            n116 = Bundle By Name(cluster=w366, "Acquisition State"=Acquisition_State."Acquiring S3DK") -> (w364:T6)
            n117 = Merge Errors(w368, w371) -> (w374:errorcluster)
          }
          frame "Idle CSV" {
          }
          frame "Acquiring CSV" {
          }
        }
      }
      frame "Acquire" {
        # "Acquire - Acquire data from the hardware. Since this is a continuous acquisition, this message will always message itself to run again."
        n118 = case shown="\"Acquiring S3DK\"" w380 {
          tunnel: [w387 w397 w399 w401] -> w386
          tunnel: w385 -> [_ w396 _ _]
          tunnel: w384 -> [w387 w392 w399 w401]
          tunnel: [w388 w394 w398 w400] -> w383
          tunnel: w382 -> [w388 w393 w398 w400]
          tunnel: w381 -> [_ w391 _ _]
          tunnel: w379 -> [_ w389 _ _]
          frame "Idle S3DK" {
            # "Ignore \"Acquire\" messages when the acquisition is idle."
          }
          frame "Acquiring S3DK" {
            # "Acquire more data while in the \"Acquiring\" state."
            n119 = call-poly "Enqueue Message.vi"("error in (no error)"=w392, "Message"=w389, "Message Queue"=w396) -> ("error out"=w390:errorcluster)  [unwired: 7 in, 1 out]
            n120 = call "Acquire.vi"("error in (no error)"=w390, "Data Queue"=w391, "Hardware Resources in"=w393) -> ("error out"=w395:errorcluster, "Hardware Resources out"=w394:T6)  [unwired: 7 in]
            n121 = Merge Errors(w395, w390) -> (w397:errorcluster)
          }
          frame "Idle CSV" {
          }
          frame "Acquiring CSV" {
          }
        }
      }
      frame "Stop" {
        # "Stop - Stop the Acquisition."
        n122 = case shown="\"Acquiring S3DK\"" w404 {
          tunnel: w407 -> [w410 w414 w419 w421]
          tunnel: [w410 w417 w419 w421] -> w406
          tunnel: w405 -> [w409 w413 w418 w420]
          tunnel: w403 -> [_ w416 _ _]
          tunnel: [w409 w412 w418 w420] -> w402
          frame "Idle S3DK" {
            # "The system is already idle. Ignore the \"Stop\" message."
          }
          frame "Acquiring S3DK" {
            # "If the system is acquiring, stop the acquisition."
            n123 = call-poly "Enqueue Message.vi"("error in (no error)"=w414, "Message"="Acquisition Stopped", "Message Queue"=w416) -> ("error out"=w417:errorcluster)  [unwired: 7 in, 1 out]
            n124 = call "Stop Acquisition.vi"("Hardware Resources in"=w413) -> ()  [unwired: 10 in, 1 out]
            n125 = Bundle By Name(cluster=w413, "Acquisition State"=Acquisition_State."Idle S3DK" ("State")) -> (w412:T6)
          }
          frame "Idle CSV" {
          }
          frame "Acquiring CSV" {
          }
        }
        n126 = Merge Errors(w406) -> (w408:errorcluster)
      }
      frame "Read Settings" {
        n127 = Send Notification(notification=w423, notifier=w422, error in (no error)=w425) -> (error out=w424:errorcluster)  [unwired: 1 out]
      }
      frame "Update Settings" {
        # "New settings are available, update the current ones stored in the shift register with the settings sent as part of the message"
        n128 = Variant To Data(error in=w428, type=w430, Variant=w433) -> (data=w431:T6, error out=w432:errorcluster)
        n129 = Select(t=w430, s=w432, f=w431) -> (s? t:f=w429:T6)
        n130 = Bundle By Name(cluster=w429, "Acquisition State"=w426) -> (w427:T6)
        n131 = Merge Errors(w428) -> (w434:errorcluster)
      }
      frame "Exit" {
        # "Stop the VI"
        # "Exit - Send the Exit message to the UI Message Handler."
        n132 = call "Shutdown S3DK.vi"("error in (no error)"=w436, "Hardware Resources in"=w438) -> ("error out"=w437:errorcluster)  [unwired: 9 in]
        n133 = Unbundle By Name(w438) -> ("Settings"=w439:string)
        n134 = call "Save Settings to XML.vim"("error in (no error)"=w437, "Settings File Name"=w439) -> ("error out"=w435:errorcluster)  [unwired: 9 in]
        n135 = Merge Errors(w435, w436) -> (w440:errorcluster)
      }
      frame "---Copy This Frame---" {
        # "Duplicate this frame when creating new messages.  Change this comment in the duplicated frame to describe this message."
        n136 = Merge Errors(w444) -> (w442:errorcluster)
      }
      frame Default {
        # "'Default' case only runs if there is a message that isn't defined in any of the other cases.  Output a programming error."
        n137 = xnode "Error Ring"("parameter 0"=w445) -> ("error out"=w446:errorcluster)
      }
    }
    n138 = call "Error Handler - Acquisition Message Loop.vi"("error in (no error)"=w333, "Message Queue"=w330) -> ("dup error in"=w323:errorcluster)  [unwired: 8 in, 1 out]
  }
  n139 = while {
    shift-right: [w465] -> w34
    shift-left: w39 -> [w466]
    tunnel: w17 -> [w459]
    shift-right: [w457] -> _
    shift-left: _ -> [w458]
    shift-right: [w463] -> w45
    shift-left: _ -> [w455]
    stop <- w464 stop-if-true
    # "Event Handling Loop"
    n140 = Not(x=w458) -> (.not. x?=w457:bool)
    "Events" <- w457
    n141 = Unbundle By Name(w459) -> ("UI"=w460:refnum<queue>)
    n142 = event shown="[1] \"Start\": Value Change" {
      selector: w466 -> [_ _ _ _ _ _ _ _ _ _]
      dyn-events: [_ _ _ _ _ _ _ _ _ _] -> w465
      timeout: 1000 -> [_ _ _ _ _ _ _ _ _ _]
      tunnel: [_ _ _ _ _ _ _ _ _ TRUE ("Discard?")] -> w464
      tunnel: w460 -> [w467 w471 w473 w477 w482 w485 w487 w494 w498 w511]
      tunnel: [_ w469 _ w476 w480 _ w490 w491 w499 _] -> w462
      tunnel: [w467 w468 w472 w475 w481 w485 w486 w494 w498 w511] -> w461
      tunnel: w455 -> [_ _ _ _ _ _ _ w492 w500 _]
      event Timeout {
        n143 = event-data() -> ()  [unwired: 1 in, 1 out]
      }
      event "Start": Value Change {
        n144 = event-data() -> ()  [unwired: 1 in, 1 out]
        n145 = call-poly "Enqueue Message.vi"("Message"="Start", "Message Queue"=w471) -> ("error out"=w469:errorcluster, "dup Message Queue"=w468:refnum<queue>)  [unwired: 8 in]
      }
      event "Settings": Value Change {
        n146 = event-data() -> ()  [unwired: 1 in, 1 out]
        n147 = call-poly "Enqueue Message.vi"("Message"="Launch Settings Dialog", "Message Queue"=w473) -> ("dup Message Queue"=w472:refnum<queue>)  [unwired: 8 in, 1 out]
      }
      event "Stop": Value Change {
        n148 = event-data() -> ()  [unwired: 1 in, 1 out]
        n149 = call-poly "Enqueue Message.vi"("Message"="Stop", "Message Queue"=w477) -> ("error out"=w476:errorcluster, "dup Message Queue"=w475:refnum<queue>)  [unwired: 8 in]
      }
      event Panel Close? {
        # "Send the 'Confirm Quit' message if the user closes the panel of the VI. Discard the event so the 'Confirm Quit' message has a chance to run."
        n150 = event-data() -> ()  [unwired: 1 in, 1 out]
        n151 = call-poly "Enqueue Message.vi"("Priority Message? (F)"=TRUE, "Message"="Confirm Quit", "Message Queue"=w482) -> ("error out"=w480:errorcluster, "dup Message Queue"=w481:refnum<queue>)  [unwired: 7 in]
        n152 = event-data("Discard?"=TRUE) -> ()  [unwired: 1 in, 1 out]
      }
      event Application Instance Close {
        n153 = event-data() -> ()  [unwired: 1 in, 1 out]
      }
      event "Exit": Value Change {
        w488 = TRUE  # Priority Message
        # "The UI Message Loop handles sending the Exit message to other loops."
        n154 = event-data() -> ()  [unwired: 1 in, 1 out]
        n155 = call-poly "Enqueue Message.vi"("Priority Message? (F)"=w488, "Message"="Exit", "Message Queue"=w487) -> ("error out"=w490:errorcluster, "dup Message Queue"=w486:refnum<queue>)  [unwired: 7 in]
      }
      event "PRL Visible": Value Change {
        n156 = event-data() -> ()  [unwired: 1 in, 1 out]
        n157 = Select(t=T16."Open Panel" ("Action"), s="PRL Visible", f=T16."Close Panel" ("Action")) -> (s? t:f=w497:T16)
        n158 = call <vilib>:"PRL Remote.vi"("error in (no error)"=w492, "Action"=w497) -> ("error out"=w491:errorcluster)  [unwired: 4 in, 5 out]
      }
      event "Data Selector": Value Change {
        n159 = event-data() -> ()  [unwired: 1 in, 1 out]
        n160 = vi-ref "S3DK.lvlib:PMU Recorder Light.lvlib:PRL Channel Selector.vi"() -> (w502:refnum<vi>)
        n161 = case shown="False" "Data Selector" {
          tunnel: w502 -> [w505 w510]
          tunnel: w500 -> [w504 w506]
          tunnel: [w503 w507] -> w499
          frame False {
            n162 = invoke class="VI" method="FP.Close"(reference=w505, error in=w504) -> (error out=w503:errorcluster)  [unwired: 1 in, 2 out]
          }
          frame True {
            n163 = invoke class="VI" method="FP.Open"(reference=w510, error in=w506, "Activate"=TRUE ("Activate?"), "State"=T17."Standard") -> (error out=w507:errorcluster)  [unwired: 1 in, 4 out]
          }
        }
      }
      event User Event {
        # "The Message Handling Loop processed an \"Exit\" message, which fired this event to stop the Event Handling Loop."
        n164 = event-data() -> ()  [unwired: 1 in, 1 out]
        n165 = local write "Status"("Exit" ("Exit String")) -> ()
      }
    }
    n166 = call "Error Handler - Event Handling Loop.vi"("error in (no error)"=w462, "Message Queue"=w461) -> ("dup error in"=w463:errorcluster)  [unwired: 8 in, 1 out]
  }
  n167 = while {
    shift-right: [w519] -> _
    shift-left: w27 -> [w521]
    tunnel: w35 -> [w518]
    tunnel: w17 -> [w515]
    shift-right: [w522] -> _
    shift-left: _ -> [w523]
    tunnel: w24 -> [w517]
    tunnel: [w518] -> w18
    tunnel: w4 -> [w516]
    tunnel: [w527] -> w3
    stop <- w532 stop-if-true
    # "Logging Loop"
    n168 = Unbundle By Name(w515) -> ("Processing"=w514:refnum<queue>, "UI"=w524:refnum<queue>, "Logging"=w525:refnum<queue>)
    n169 = Unbundle By Name(w521) -> ("Logging State"=w520:T5)
    n170 = Not(x=w523) -> (.not. x?=w522:bool)
    "Buffer" <- w522
    n171 = call "Dequeue Message.vi"("error in (no error)"=w516, "Message Queue"=w525) -> ("error out"=w531:errorcluster, "Message Data"=w529:variant, "Message"=w530:string, "dup Message Queue"=w528:refnum<queue>)  [unwired: 6 in]
    n172 = case "Message Cases" shown="\"Exit\"" w530 {
      selector: w530 -> [_ w552 _ _ _ _ _ _ w646]
      tunnel: w528 -> [_ w557 w573 _ _ _ _ _ _]
      tunnel: w531 -> [w538 w551 w571 w597 w623 w626 w639 w645 _]
      tunnel: [w539 w558 w574 w600 w622 w632 w641 w643 w647] -> w526
      tunnel: w521 -> [w540 w556 w570 w594 w621 w630 w636 w644 w648]
      tunnel: [w549 w555 w570 w593 w621 w625 w636 w644 w648] -> w519
      tunnel: [_ _ _ _ _ _ TRUE _ _] -> w532
      tunnel: w529 -> [_ _ _ _ _ w631 _ _ _]
      tunnel: w524 -> [_ _ _ w595 _ _ _ _ _]
      tunnel: w518 -> [_ _ w572 w598 _ _ w640 _ _]
      tunnel: w520 -> [_ w554 w569 w596 _ w624 _ _ _]
      tunnel: w517 -> [_ _ _ _ w620 _ _ _ _]
      tunnel: w514 -> [_ w553 _ _ _ _ _ _ _]
      frame "Initialize" {
        w543 = T15 2 items=["no dialog", "OK message", "continue or stop message", "OK message + warnings", "continue/stop + warnings"] ("type of dialog (OK msg:1)")
        # "Initialize - gets called when first launched. Currently a no-op."
        n173 = Unbundle By Name(w540) -> ("Settings"=w546:string)
        n174 = call "Load Settings from XML.vim"("error in (no error)"=w538, "Settings File Name"=w546, "Settings In"=w540) -> ("error out"=w544:errorcluster, "Settings Out"=w545:T4)  [unwired: 7 in]
        n175 = Variant To Data(error in=w544, type=w540, Variant=w545) -> (data=w541:T4, error out=w534:errorcluster)
        n176 = Select(t=w540, s=w534, f=w541) -> (s? t:f=w536:T4)
        n177 = Unbundle By Name(w536) -> ("Buffer"=w535:T3)
        n178 = call "Buffer.vi"("Parameters"=w535, "Mode"=Buffer_state."Init", "Error IN"=w534) -> ("Error OUT"=w533:errorcluster)  [unwired: 4 in, 4 out]
        n179 = call <vilib>:"General Error Handler.vi"("[error source] (\" \")"="Log. Settings" ("[error source] (\" \")"), "type of dialog (OK msg:1)"=w543, "error in (no error)"=w533) -> ("error out"=w539:errorcluster)  [unwired: 8 in, 4 out]
        n180 = Bundle By Name(cluster=w536, "Logging State"=Logging_State."Idle" ("State"), "Settings"="Logging") -> (w549:T4)
      }
      frame "Start" {
        # "Start - Send the \"Log\" message to start logging.  Generate a unique, timestamped TDMS file name based on the Log File Base Path value."
        n181 = call-poly "Enqueue Message.vi"("error in (no error)"=w551, "Message"=w552, "Message Queue"=w553) -> ("error out"=w550:errorcluster)  [unwired: 7 in, 1 out]
        n182 = case shown="\"Idle\"" w554 {
          tunnel: [w559 w564] -> w558
          tunnel: w557 -> [_ w565]
          tunnel: w550 -> [w559 w563]
          tunnel: w556 -> [w560 w566]
          tunnel: [w560 w567] -> w555
          frame "Logging" {
            # "The system is already logging. Ignore the \"Start\" message."
          }
          frame "Idle" {
            # "If the system is idle, start logging."
            n183 = call-poly "Enqueue Message.vi"("error in (no error)"=w563, "Message"="Log", "Message Queue"=w565) -> ("error out"=w561:errorcluster)  [unwired: 7 in, 1 out]
            n184 = Merge Errors(w561) -> (w564:errorcluster)
            n185 = Bundle By Name(cluster=w566, "Logging State"=Logging_State."Logging" ("State")) -> (w567:T4)
          }
        }
      }
      frame "Log" {
        # "Log - Log data to disk. Since this is a continuous acquisition, this message will always message itself to run again."
        n186 = case shown="\"Logging\"" w569 {
          tunnel: [w575 w587] -> w574
          tunnel: w573 -> [_ w586]
          tunnel: w572 -> [_ w583]
          tunnel: w571 -> [w575 w584]
          frame "Idle" {
            # "Ignore \"Log\" messages when the logging is idle."
          }
          frame "Logging" {
            # "Throttling to a minimum\nof 15 ms in the loop"
            # "Log more data while in the \"Logging\" state."
            n187 = call-poly "Enqueue Message.vi"("error in (no error)"=w584, "Message"="Log", "Message Queue"=w586) -> ("error out"=w581:errorcluster)  [unwired: 7 in, 1 out]
            n188 = Dequeue Element(queue=w583, timeout in ms (-1)=40, error in (no error)=w581) -> (element=w578:T9[], timed out?=w580:bool, error out=w579:errorcluster)  [unwired: 1 out]
            n189 = case shown="False" w580 {
              tunnel: w579 -> [w590 w592]
              tunnel: w578 -> [w591 _]
              tunnel: [w588 w592] -> w577
              frame False {
                n190 = call "Buffer.vi"("Mode"=Buffer_state."Add", "Error IN"=w590, "DATA IN"=w591) -> ("Error OUT"=w588:errorcluster)  [unwired: 4 in, 4 out]
              }
              frame True {
              }
            }
            n191 = Merge Errors(w577, w581) -> (w587:errorcluster)
            n192 = Wait Until Next ms Multiple(millisecond multiple=u32 15) -> ()  [unwired: 1 out]
          }
        }
      }
      frame "Stop" {
        # "Stop - Flush the message queue of any pending \"Log\" messages. Call 'Flush Data to Log File.vi' so any pending data is not lost."
        n193 = case shown="\"Logging\"" w596 {
          tunnel: [w602 w614] -> w599
          tunnel: w598 -> [_ w607]
          tunnel: w597 -> [w602 w608]
          tunnel: w595 -> [_ w613]
          tunnel: w594 -> [w601 w609]
          tunnel: [w601 w611] -> w593
          frame "Idle" {
            # "The system is already idle. Ignore the \"Stop\"."
          }
          frame "Logging" {
            # "If the system is logging, stop logging."
            n194 = Flush Queue(queue=w607, error in (no error)=w608) -> (remaining elements=w606:cluster{T9[]}[], error out=w605:errorcluster)  [unwired: 1 out]
            n195 = for {
              tunnel: w606 -> [w619] mode=indexing
              shift-right: [w617] -> w603
              shift-left: w605 -> [w616]
              tunnel: Buffer_state."Add" ("Mode") -> [w615]
              n196 = Unbundle(w619) -> (w618:T9[])
              n197 = call "Buffer.vi"("Mode"=w615, "Error IN"=w616, "DATA IN"=w618) -> ("Error OUT"=w617:errorcluster)  [unwired: 4 in, 4 out]
            }
            n198 = Bundle By Name(cluster=w609, "Logging State"=Logging_State."Idle" ("State")) -> (w611:T4)
            n199 = call-poly "Enqueue Message.vi"("error in (no error)"=w603, "Message"="Logging Stopped", "Message Queue"=w613) -> ("error out"=w614:errorcluster)  [unwired: 7 in, 1 out]
          }
        }
        n200 = Merge Errors(w599) -> (w600:errorcluster)
      }
      frame "Read Settings" {
        n201 = Send Notification(notification=w621, notifier=w620, error in (no error)=w623) -> (error out=w622:errorcluster)  [unwired: 1 out]
      }
      frame "Update Settings" {
        # "Update Settings - New settings are available, update the current ones stored in the shift register with the settings sent as part of the message."
        n202 = Variant To Data(error in=w626, type=w630, Variant=w631) -> (data=w629:T4, error out=w628:errorcluster)
        n203 = Select(t=w630, s=w628, f=w629) -> (s? t:f=w627:T4)
        n204 = Merge Errors(w626) -> (w632:errorcluster)
        n205 = Bundle By Name(cluster=w627, "Logging State"=w624) -> (w625:T4)
      }
      frame "Exit" {
        # "Stop the VI"
        # "Exit - Send the Exit message to the UI Message Handler.  Call 'Flush Data to Log File.vi' so any pending data is not lost."
        n206 = Flush Queue(queue=w640, error in (no error)=w639) -> (error out=w638:errorcluster)  [unwired: 2 out]
        n207 = call "Buffer.vi"("Mode"=Buffer_state."Exit", "Error IN"=w638) -> ("Error OUT"=w634:errorcluster)  [unwired: 5 in, 4 out]
        n208 = Unbundle By Name(w636) -> ("Settings"=w635:string)
        n209 = call "Save Settings to XML.vim"("error in (no error)"=w634, "Settings File Name"=w635, "Settings In"=w636) -> ("error out"=w633:errorcluster)  [unwired: 8 in]
        n210 = Merge Errors(w633, w639) -> (w641:errorcluster)
      }
      frame "---Copy This Frame---" {
        # "Duplicate this frame when creating new messages.  Change this comment in the duplicated frame to describe this message."
        n211 = Merge Errors(w645) -> (w643:errorcluster)
      }
      frame Default {
        # "'Default' case only runs if there is a message that isn't defined in any of the other cases.  Output a programming error."
        n212 = xnode "Error Ring"("parameter 0"=w646) -> ("error out"=w647:errorcluster)
      }
    }
    n213 = call "Error Handler - Logging Message Loop.vi"("error in (no error)"=w526, "Message Queue"=w524) -> ("dup error in"=w527:errorcluster)  [unwired: 8 in, 1 out]
  }
  n214 = while {
    tunnel: w29 -> [w660]
    shift-right: [w672] -> _
    shift-left: _ -> [w671]
    tunnel: w23 -> [w659]
    shift-right: [w662] -> _
    shift-left: w26 -> [w663]
    tunnel: w17 -> [w669]
    tunnel: w4 -> [w668]
    tunnel: [w657] -> w2
    stop <- w661 stop-if-true
    # "Algorithm Loop"
    n215 = Unbundle By Name(w669) -> ("UI"=w656:refnum<queue>, "Processing"=w670:refnum<queue>)
    n216 = Not(x=w671) -> (.not. x?=w672:bool)
    "Processing" <- w672
    n217 = call "Dequeue Message.vi"("error in (no error)"=w668, "Message Queue"=w670) -> ("error out"=w665:errorcluster, "Message Data"=w664:variant, "Message"=w666:string, "dup Message Queue"=w667:refnum<queue>)  [unwired: 6 in]
    n218 = case "Message Cases" shown="\"Process\"" w666 {
      selector: w666 -> [_ _ w709 _ _ _ _ _ w744]
      tunnel: w667 -> [_ w690 w708 w716 _ _ _ _ _]
      tunnel: w665 -> [w678 w692 w710 w717 w723 w726 w731 w742 _]
      tunnel: w663 -> [w680 w693 w705 w719 w720 w729 w733 w741 w745]
      tunnel: [w688 w693 w705 w719 w720 w725 w733 w741 w745] -> w662
      tunnel: [_ _ _ _ _ _ TRUE _ _] -> w661
      tunnel: w664 -> [_ _ _ _ _ w730 _ _ _]
      tunnel: [w677 w691 w707 w718 w722 w724 w738 w740 w743] -> w658
      tunnel: w660 -> [_ _ w699 _ _ _ w737 _ _]
      tunnel: w659 -> [_ _ _ _ w721 _ _ _ _]
      frame "Initialize" {
        w683 = T15 2 items=["no dialog", "OK message", "continue or stop message", "OK message + warnings", "continue/stop + warnings"] ("type of dialog (OK msg:1)")
        # "Initialize - gets called when first launched. Currently a no-op."
        n219 = Unbundle By Name(w680) -> ("Settings"=w686:string)
        n220 = call "Load Settings from XML.vim"("error in (no error)"=w678, "Settings File Name"=w686, "Settings In"=w680) -> ("error out"=w684:errorcluster, "Settings Out"=w685:T2)  [unwired: 7 in]
        n221 = Variant To Data(error in=w684, type=w680, Variant=w685) -> (data=w681:T2, error out=w676:errorcluster)
        n222 = Select(t=w680, s=w676, f=w681) -> (s? t:f=w679:T2)
        n223 = call "Buffer.vi"("Mode"=Buffer_state."Add_Serv", "Error IN"=w676) -> ("Error OUT"=w673:errorcluster, "Index"=w675:i32)  [unwired: 5 in, 3 out]
        n224 = call <vilib>:"General Error Handler.vi"("[error source] (\" \")"="Proc. Settings" ("[error source] (\" \")"), "type of dialog (OK msg:1)"=w683, "error in (no error)"=w673) -> ("error out"=w677:errorcluster)  [unwired: 8 in, 4 out]
        n225 = Bundle By Name(cluster=w679, "Settings"="Processing", "Parameters.Index"=w675) -> (w688:T2)
      }
      frame "Start" {
        # "Start - Send the \"Log\" message to start logging.  Generate a unique, timestamped TDMS file name based on the Log File Base Path value."
        n226 = call-poly "Enqueue Message.vi"("error in (no error)"=w692, "Message"="Process", "Message Queue"=w690) -> ("error out"=w691:errorcluster)  [unwired: 7 in, 1 out]
      }
      frame "Process" {
        n227 = Unbundle By Name(w705) -> ("Parameters"=w704:T3)
        n228 = call-poly "Enqueue Message.vi"("error in (no error)"=w710, "Message"=w709, "Message Queue"=w708) -> ("error out"=w707:errorcluster)  [unwired: 7 in, 1 out]
        n229 = Bundle By Name(cluster=w704, "Size"=0, "Ordered ?"=TRUE) -> (w703:T3)
        n230 = call "Buffer.vi"("Parameters"=w703, "Mode"=Buffer_state."Get", "Error IN"=w707) -> ("Output"=w700:T19, "New Element ?"=w694:bool)  [unwired: 4 in, 3 out]
        n231 = Unbundle By Name(w700) -> ("Analog"=w698:sgl[][])
        n232 = Index Array(array=w698, index (col)=0 ("disabled index (col)")) -> (element=w696:sgl[])  [unwired: 1 in]
        n233 = case shown="True" w694 {
          tunnel: w699 -> [_ w714]
          tunnel: w696 -> [_ w712]
          frame False {
          }
          frame True {
            n234 = Bundle By Name(cluster=T1 {"Data"=[]} ("Display Data"), "Data"=w712) -> (w713:T1)
            n235 = Send Notification(notification=w713, notifier=w714) -> ()  [unwired: 1 in, 2 out]
          }
        }
        n236 = Wait Until Next ms Multiple(millisecond multiple=u32 500) -> ()  [unwired: 1 out]
      }
      frame "Stop" {
        # "Stop - Flush the message queue of any pending \"Log\" messages. Call 'Flush Data to Log File.vi' so any pending data is not lost."
        n237 = Flush Queue(queue=w716, error in (no error)=w717) -> (error out=w715:errorcluster)  [unwired: 2 out]
        n238 = Merge Errors(w715) -> (w718:errorcluster)
      }
      frame "Read Settings" {
        n239 = Send Notification(notification=w720, notifier=w721, error in (no error)=w723) -> (error out=w722:errorcluster)  [unwired: 1 out]
      }
      frame "Update Settings" {
        # "Update Settings - New settings are available, update the current ones stored in the shift register"
        n240 = Variant To Data(error in=w726, type=w729, Variant=w730) -> (data=w728:T2, error out=w727:errorcluster)
        n241 = Select(t=w729, s=w727, f=w728) -> (s? t:f=w725:T2)
        n242 = Merge Errors(w726) -> (w724:errorcluster)
      }
      frame "Exit" {
        # "Stop the VI"
        # "Exit - Send the Exit message to the UI Message Handler.  Call 'Flush Data to Log File.vi' so any pending data is not lost."
        n243 = Release Notifier(notifier=w737, force destroy? (F)=TRUE, error in (no error)=w731) -> (error out=w736:errorcluster)  [unwired: 2 out]
        n244 = Unbundle By Name(w733) -> ("Settings"=w734:string)
        n245 = call "Save Settings to XML.vim"("error in (no error)"=w731, "Settings File Name"=w734, "Settings In"=w733) -> ("error out"=w732:errorcluster)  [unwired: 8 in]
        n246 = Merge Errors(w732, w736) -> (w738:errorcluster)
      }
      frame "---Copy This Frame---" {
        # "Duplicate this frame when creating new messages.  Change this comment in the duplicated frame to describe this message."
        n247 = Merge Errors(w742) -> (w740:errorcluster)
      }
      frame Default {
        # "'Default' case only runs if there is a message that isn't defined in any of the other cases.  Output a programming error."
        n248 = xnode "Error Ring"("parameter 0"=w744) -> ("error out"=w743:errorcluster)
      }
    }
    n249 = call "Error Handler - Processing Message Loop.vi"("error in (no error)"=w658, "Message Queue"=w656) -> ("dup error in"=w657:errorcluster)  [unwired: 8 in, 1 out]
  }
  n250 = Unregister For Events(event registration refnum=w34, error in=w45) -> (error out=w43:errorcluster)
  n251 = Merge Errors(w43, w33, w5, w3, w2) -> (w32:errorcluster)
  n252 = call "Destroy User Event - Stop.vi"("error in (no error)"=w32, "User Event - Stop"=w38) -> ("error out"=w30:errorcluster)  [unwired: 9 in]
  n253 = Cluster To Array(cluster=w16) -> (array=w31:refnum<queue>[])
  n254 = for {
    shift-right: [w756] -> w7
    shift-left: w30 -> [w755]
    tunnel: w6 -> [w754]
    tunnel: w31 -> [w753] mode=indexing
    n255 = Release Queue(queue=w753, force destroy? (F)=w754, error in (no error)=w755) -> (error out=w756:errorcluster)  [unwired: 2 out]
  }
  n256 = Unbundle(w12) -> ("notifier out"=w11:refnum<notifier>, "notifier out"=w10:refnum<notifier>, "notifier out"=w9:refnum<notifier>)
  n257 = Release Notifier(notifier=w11, force destroy? (F)=w6, error in (no error)=w7) -> (error out=w14:errorcluster)  [unwired: 2 out]
  n258 = Release Notifier(notifier=w10, force destroy? (F)=w6, error in (no error)=w14) -> (error out=w13:errorcluster)  [unwired: 2 out]
  n259 = Release Notifier(notifier=w9, force destroy? (F)=w6, error in (no error)=w13) -> (error out=w8:errorcluster)  [unwired: 2 out]
  n260 = Release Queue(queue=w18, force destroy? (F)=w6, error in (no error)=w8) -> (error out=w15:errorcluster)  [unwired: 2 out]
  n261 = disable-structure shown="RUN_TIME_ENGINE==True" {
    disable-tunnel: w15 -> [_ _]
    frame condition #0 (active) {
    }
    frame condition #1 {
      # "Call Quit LabVIEW if running as a built application."
      n262 = Quit LabVIEW() -> ()  [unwired: 1 in]
    }
  }
